vi "Swing-up_Python_Simulation Data_LabVIEW_DIP_Elyes_KHECHINE_Ayoub_HEDFI_Elyes_CHAMEKH.vi"() -> ()   [LabVIEW 2022 SP3]
uses:
  <vilib>/Utility/file.llb/Read Delimited Spreadsheet (string).vi
  shell32.dll
panel:
  out "q2dot(t): Long Pendulum Joint Velocity":cluster{"Array":dbl[], "Array":dbl[]}(graph)
  out "q2dot[t]":dbl[][](array[numeric])
  out "q1dot(t): Short Pendulum Joint Velocity":cluster{"Array":dbl[], "Array":dbl[]}(graph)
  out "q1dot[t]":dbl[][](array[numeric])
  out "xdot(t): Cart velocity":cluster{"Array":dbl[], "Array":dbl[]}(graph)
  out "xdot[t]":dbl[][](array[numeric])
  out "Path":path
  out "error out":errorcluster
  in  "error in (no error)":errorcluster
  in  "Select where you saved the U.csv  simulation data file is in your system":i32(ring) items=["Desktop"=0, "Personal Documents"=5, "AppData"=26, "Local AppData"=28, "Common AppData"=35, "Program Files"=38, "Program Files Common"=43, "Common Documents"=46]
  out "q2(t): Long Pendulum Angle (deg)":cluster{"Array":dbl[], "Array":dbl[]}(graph)
  out "q1(t): Short Pendulum Angle (deg)":cluster{"Array":dbl[], "Array":dbl[]}(graph)
  out "x(t): Cart Position (mm)":cluster{"Array":dbl[], "Array":dbl[]}(graph)
  out "u(t): Motor Voltage (V)":cluster{"Array":dbl[], "Array":dbl[]}(graph)
  out "q2[t]":dbl[][](array[numeric])
  out "q1[t]":dbl[][](array[numeric])
  out "x[t]":dbl[][](array[numeric])
  out "u[t]":dbl[][](array[numeric])
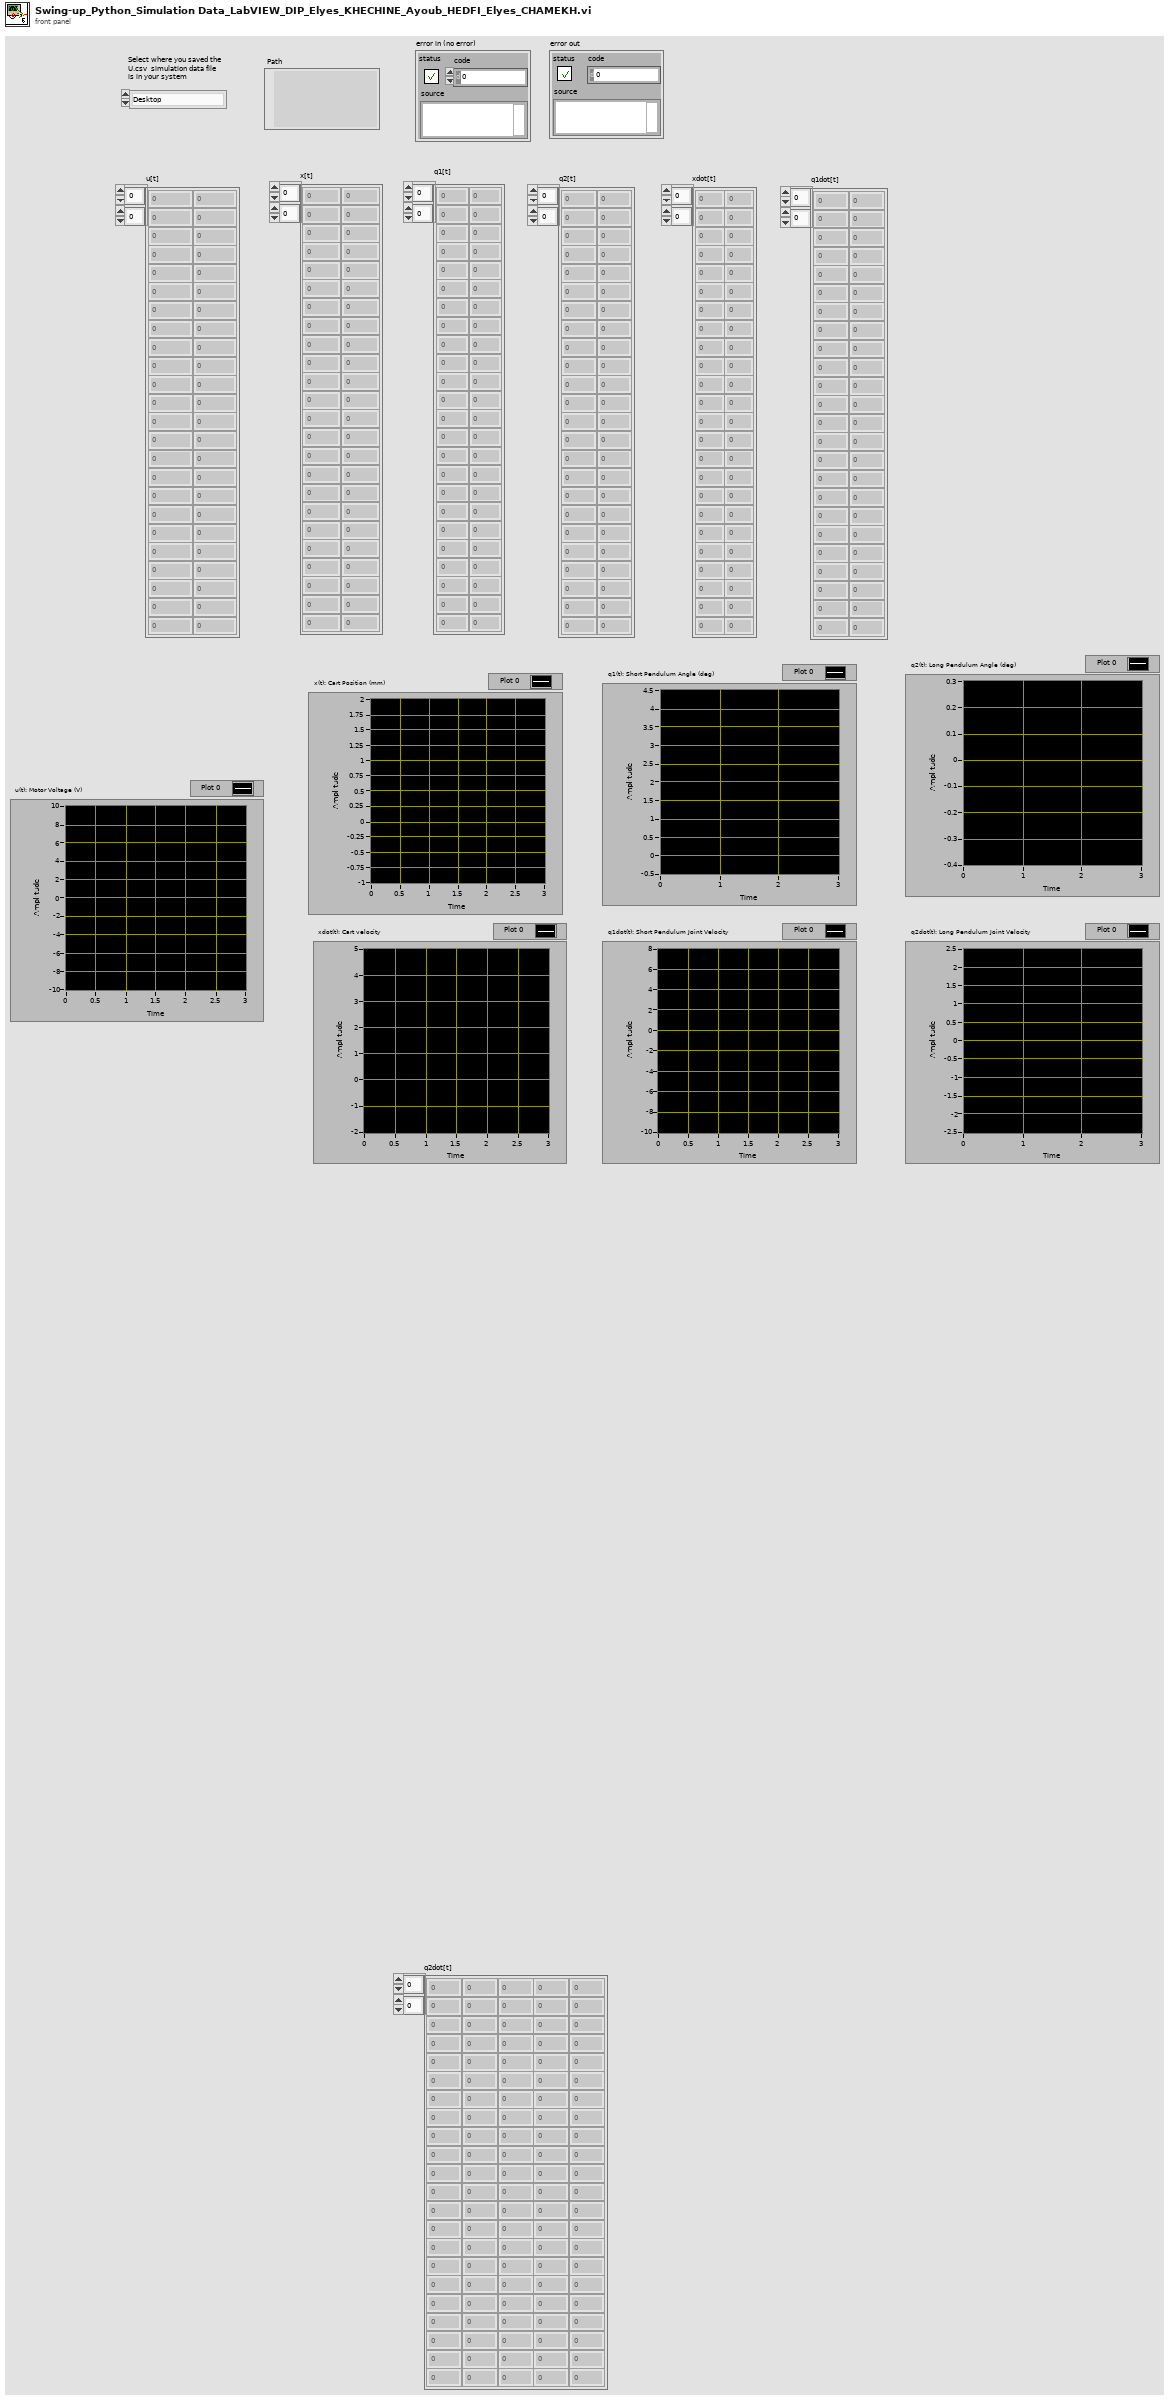
[diagram p1: front panel]
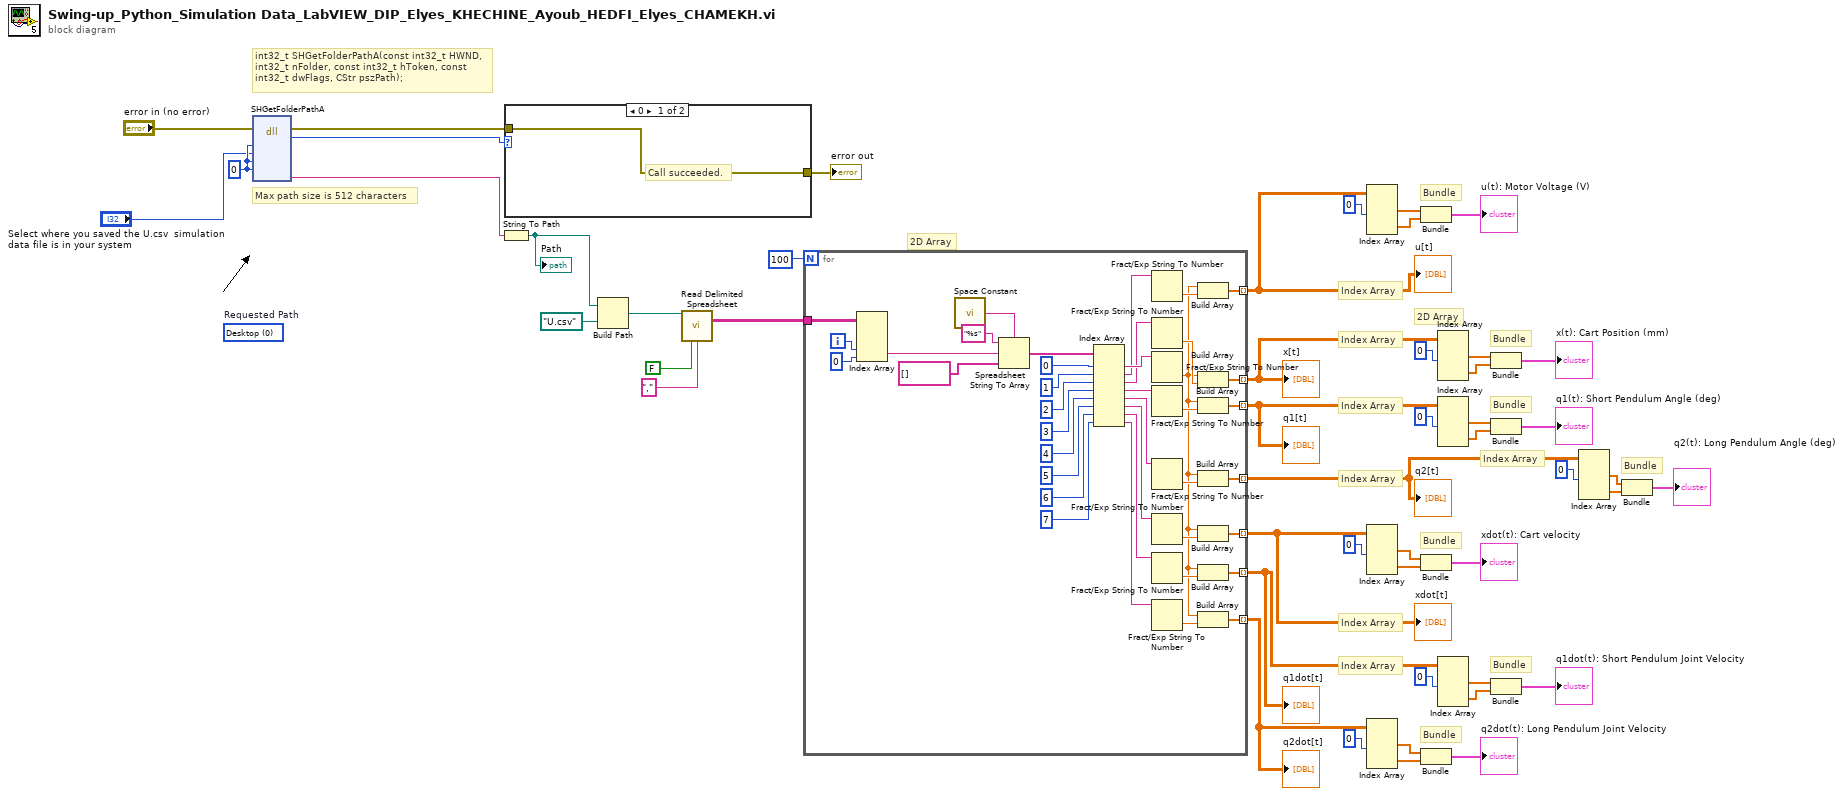
[diagram p0: block diagram]
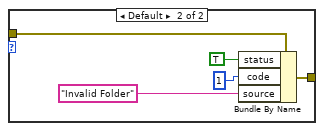
[diagram p2: hidden frame]
diagram:
  (unwired) 0 items=["Desktop"=0, "Personal Documents"=5, "AppData"=26, "Local AppData"=28, "Common AppData"=35, "Program Files"=38, "Program Files Common"=43, "Common Documents"=46]  # Requested Path
  w23 = 0 ("HWND")
  # "Index Array"
  # "Bundle"
  # "Index Array"
  # "Bundle"
  # "Index Array"
  # "Bundle"
  # "int32_t SHGetFolderPathA(const int32_t HWND, int32_t nFolder, const int32_t hToken, const int32_t dwFlags, CStr pszPath);"
  # "Max path size is 512 characters"
  # "Index Array"
  # "Bundle"
  # "Index Array"
  # "Bundle"
  # "Index Array"
  # "Bundle"
  # "2D Array"
  # "Index Array"
  # "Bundle"
  # "2D Array"
  n1 = dll-call lib="shell32.dll" fn="SHGetFolderPathA"(error in="error in (no error)", "HWND"=w23, "nFolder"="Select where you saved the U.csv  simulation data file is in your system", "hToken"=w23, "dwFlags"=w23) -> (error out=w21:errorcluster, "Succeeded"=w22:i32, "pszPath"=w24:string)  [unwired: 7 in, 1 out]
  n2 = String To Path(string=w24) -> (path=w18:path)
  "Path" <- w18
  n3 = case shown="0" w22 {
    tunnel: w21 -> [w50 w55]
    tunnel: [w50 w51] -> w20
    frame 0 {
      # "Call succeeded."
    }
    frame Default {
      n4 = Bundle By Name(cluster=w55, "status"=TRUE, "code"=1, "source"="Invalid Folder") -> (w51:errorcluster)
    }
  }
  "error out" <- w20
  n5 = Build Path(base path=w18, name or relative path=path "U.csv" ("CSV Data file path")) -> (appended path=w16:path)
  n6 = call-poly <vilib>:"Read Delimited Spreadsheet.vi"("file path (dialog if empty)"=w16, "transpose? (F)"=FALSE, "delimiter (\\t)"="," ("delimiter (\\t)")) -> ("all rows"=w46:string[][])  [unwired: 7 in, 5 out]
  n7 = for {
    N: 100 -> [_]
    tunnel: [w76] -> w41 mode=indexing
    tunnel: [w75] -> w28 mode=indexing
    tunnel: [w74] -> w27 mode=indexing
    tunnel: [w73] -> w26 mode=indexing
    tunnel: w46 -> [w72]
    tunnel: [w58] -> w11 mode=indexing
    tunnel: [w57] -> w6 mode=indexing
    tunnel: [w56] -> w1 mode=indexing
    i -> [w71]
    n8 = Index Array(array=w72, index (row) #2=w71, index (col) #2=0) -> (element #2=w69:string)  [unwired: 2 in, 1 out]
    n9 = call <vilib>:"Space Constant.vi"() -> ("String"=w92:string)
    n10 = Spreadsheet String To Array(delimiter (Tab)=w92, format string="%s", spreadsheet string=w69, array type (2D Dbl)=string[] []) -> (array=w91:string[])
    n11 = Index Array(array=w91, index #1=0, index #2=1, index #3=2, index #4=3, index #5=4, index #6=5, index #7=6, index #8=7) -> (element #1=w85:string, element #2=w84:string, element #3=w83:string, element #4=w82:string, element #5=w81:string, element #6=w63:string, element #7=w62:string, element #8=w61:string)
    n12 = Fract/Exp String To Number(string=w84) -> (number=w80:dbl)  [unwired: 3 in, 1 out]
    n13 = Fract/Exp String To Number(string=w83) -> (number=w79:dbl)  [unwired: 3 in, 1 out]
    n14 = Fract/Exp String To Number(string=w85) -> (number=w59:dbl)  [unwired: 3 in, 1 out]
    n15 = Fract/Exp String To Number(string=w82) -> (number=w78:dbl)  [unwired: 3 in, 1 out]
    n16 = Fract/Exp String To Number(string=w81) -> (number=w77:dbl)  [unwired: 3 in, 1 out]
    n17 = Fract/Exp String To Number(string=w63) -> (number=w65:dbl)  [unwired: 3 in, 1 out]
    n18 = Fract/Exp String To Number(string=w62) -> (number=w64:dbl)  [unwired: 3 in, 1 out]
    n19 = Fract/Exp String To Number(string=w61) -> (number=w60:dbl)  [unwired: 3 in, 1 out]
    n20 = Build Array(w59, w80) -> (w76:dbl[])
    n21 = Build Array(w59, w79) -> (w75:dbl[])
    n22 = Build Array(w59, w78) -> (w74:dbl[])
    n23 = Build Array(w59, w77) -> (w73:dbl[])
    n24 = Build Array(w59, w65) -> (w58:dbl[])
    n25 = Build Array(w59, w64) -> (w57:dbl[])
    n26 = Build Array(w59, w60) -> (w56:dbl[])
  }
  "u[t]" <- w41
  "x[t]" <- w28
  "q1[t]" <- w27
  "q2[t]" <- w26
  "xdot[t]" <- w11
  "q1dot[t]" <- w6
  "q2dot[t]" <- w1
  n27 = Index Array(array=w41, index (col) #1=0 ("disabled index (col)")) -> (element #1=w42:dbl[], element #2=w43:dbl[])  [unwired: 3 in]
  n28 = Index Array(array=w11, index (col) #1=0 ("disabled index (col)")) -> (element #1=w12:dbl[], element #2=w13:dbl[])  [unwired: 3 in]
  n29 = Index Array(array=w1, index (col) #1=0 ("disabled index (col)")) -> (element #1=w2:dbl[], element #2=w3:dbl[])  [unwired: 3 in]
  n30 = Bundle(w42, w43) -> (→"u(t): Motor Voltage (V)":cluster{dbl[], dbl[]})  [unwired: 1 in]
  n31 = Bundle(w12, w13) -> (→"xdot(t): Cart velocity":cluster{dbl[], dbl[]})  [unwired: 1 in]
  n32 = Bundle(w2, w3) -> (→"q2dot(t): Long Pendulum Joint Velocity":cluster{dbl[], dbl[]})  [unwired: 1 in]
  n33 = Index Array(array=w28, index (col) #1=0 ("disabled index (col)")) -> (element #1=w37:dbl[], element #2=w38:dbl[])  [unwired: 3 in]
  n34 = Index Array(array=w27, index (col) #1=0 ("disabled index (col)")) -> (element #1=w33:dbl[], element #2=w34:dbl[])  [unwired: 3 in]
  n35 = Index Array(array=w6, index (col) #1=0 ("disabled index (col)")) -> (element #1=w7:dbl[], element #2=w8:dbl[])  [unwired: 3 in]
  n36 = Bundle(w37, w38) -> (→"x(t): Cart Position (mm)":cluster{dbl[], dbl[]})  [unwired: 1 in]
  n37 = Bundle(w33, w34) -> (→"q1(t): Short Pendulum Angle (deg)":cluster{dbl[], dbl[]})  [unwired: 1 in]
  n38 = Bundle(w7, w8) -> (→"q1dot(t): Short Pendulum Joint Velocity":cluster{dbl[], dbl[]})  [unwired: 1 in]
  n39 = Index Array(array=w26, index (col) #1=0 ("disabled index (col)")) -> (element #1=w29:dbl[], element #2=w30:dbl[])  [unwired: 3 in]
  n40 = Bundle(w29, w30) -> (→"q2(t): Long Pendulum Angle (deg)":cluster{dbl[], dbl[]})  [unwired: 1 in]
